vi "updateValues.vi"(8 "error in (no error)":errorcluster, 11 "Rf_Ramp_Action in":refnum<class "Rf_Ramp_Action.lvclass">) -> (0 "error out":errorcluster, 3 "Rf_Ramp_Action out":refnum<class "Rf_Ramp_Action.lvclass">)   [LabVIEW 2011, in "Views.lvlib" / "ScriptEditor.lvlib" / "Rf_Ramp_Action.lvclass"]
uses:
  Rf_Ramp_Action.lvclass
  Tools/Scripting/ScriptingEvent/ScriptEvents/RfRamp/RfRamp.lvclass
  Rf_Ramp_Action.lvclass/Rf_Ramp_Action.ctl
  Tools/Scripting/ScriptingEvent/ScriptEvent.lvclass
  Tools/Scripting/ScriptingEvent/ScriptEvents/Rf Event/rf.lvclass
  ActionPanel.lvclass
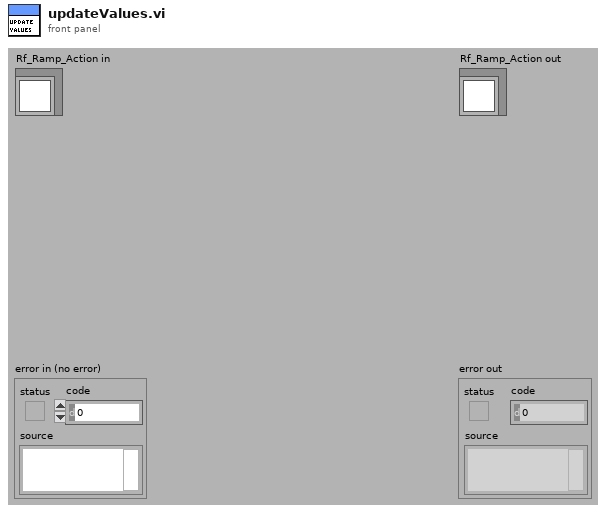
[diagram p1: front panel]
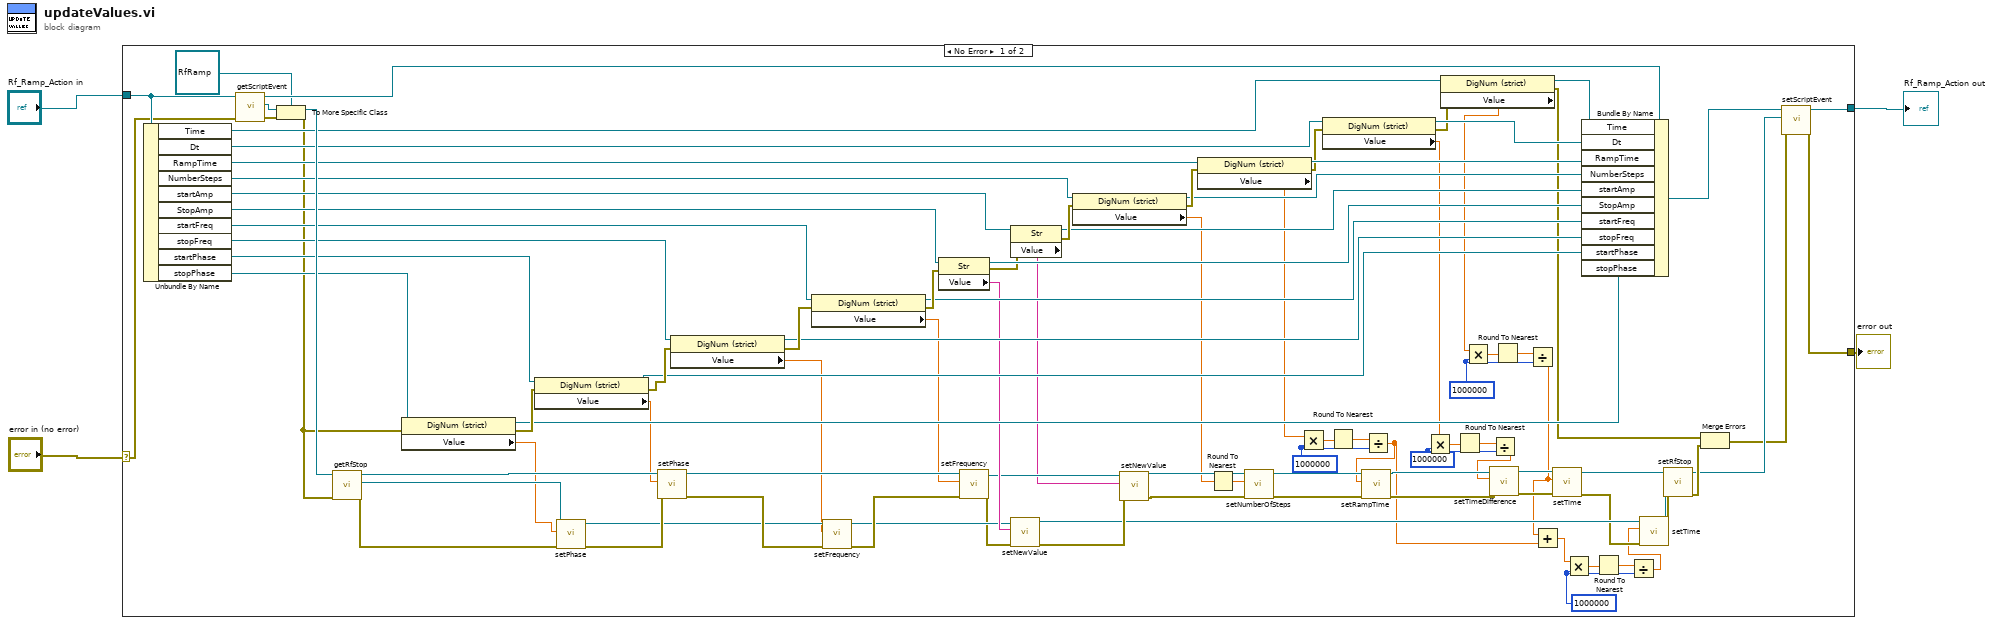
[diagram p0: block diagram]
diagram:
  n1 = case shown="No Error" "error in (no error)" {
    selector: "error in (no error)" -> [w100 w103]
    tunnel: [w27 w103] -> w3
    tunnel: [w29 w102] -> w1
    tunnel: "Rf_Ramp_Action in" -> [w101 w102]
    frame No Error {
      w7 = 1000000
      w12 = 1000000
      w17 = 1000000
      w22 = 1000000
      n2 = Unbundle By Name(w101) -> ("Time"=w67:refnum<vi>, "Dt"=w70:refnum<vi>, "RampTime"=w72:refnum<vi>, "NumberSteps"=w73:refnum<vi>, "startAmp"=w75:refnum<vi>, "StopAmp"=w78:refnum<vi>, "startFreq"=w79:refnum<vi>, "stopFreq"=w80:refnum<vi>, "startPhase"=w81:refnum<vi>, "stopPhase"=w82:refnum<vi>)
      n3 = call "getScriptEvent.vi"("error in (no error)"=w100, "ActionPanel.lvclass in"=w101) -> ("error out"=w84:errorcluster, "ScriptEvent.lvclass"=w86:refnum<class "ScriptEvent.lvclass">, "ActionPanel.lvclass out"=w87:refnum<class "Rf_Ramp_Action.lvclass">)  [unwired: 7 in]
      n4 = To More Specific Class(target class=refnum<class "RfRamp.lvclass"> refnum ("RfRamp out"), reference=w86, error in=w84) -> (specific class reference=w83:refnum<class "RfRamp.lvclass">, error out=w61:errorcluster)
      n5 = call "getRfStop.vi"("error in (no error)"=w61, "RfRamp in"=w83) -> ("error out"=w62:errorcluster, "rfStop"=w66:refnum<class "rf.lvclass">, "RfRamp out"=w65:refnum<class "RfRamp.lvclass">)  [unwired: 7 in]
      n6 = property class="DigNum (strict)"(reference=w82, error in=w61) -> (reference out=w88:refnum<vi>, error out=w89:errorcluster, "Value"=w26:dbl)
      n7 = property class="DigNum (strict)"(reference=w81, error in=w89) -> (reference out=w90:refnum<vi>, error out=w99:errorcluster, "Value"=w64:dbl)
      n8 = call "setPhase.vi"("error in (no error)"=w62, "phase"=w26, "rf in"=w66) -> ("error out"=w63:errorcluster, "rf out"=w57:refnum<class "rf.lvclass">)  [unwired: 7 in]
      n9 = call "setPhase.vi"("error in (no error)"=w63, "phase"=w64, "rf in"=w65) -> ("error out"=w58:errorcluster, "rf out"=w60:refnum<class "RfRamp.lvclass">)  [unwired: 7 in]
      n10 = property class="DigNum (strict)"(reference=w80, error in=w99) -> (reference out=w91:refnum<vi>, error out=w98:errorcluster, "Value"=w56:dbl)
      n11 = property class="DigNum (strict)"(reference=w79, error in=w98) -> (reference out=w92:refnum<vi>, error out=w97:errorcluster, "Value"=w55:dbl)
      n12 = call "setFrequency.vi"("error in (no error)"=w58, "frequency"=w56, "rf in"=w57) -> ("error out"=w59:errorcluster, "rf out"=w53:refnum<class "rf.lvclass">)  [unwired: 7 in]
      n13 = property class="Str"(reference=w78, error in=w97) -> (reference out=w93:refnum<vi>, error out=w76:errorcluster, "Value"=w54:string)
      n14 = call "setFrequency.vi"("error in (no error)"=w59, "frequency"=w55, "rf in"=w60) -> ("error out"=w52:errorcluster, "rf out"=w51:refnum<class "RfRamp.lvclass">)  [unwired: 7 in]
      n15 = property class="Str"(reference=w75, error in=w76) -> (reference out=w74:refnum<vi>, error out=w77:errorcluster, "Value"=w49:string)
      n16 = call "setNewValue.vi"("error in (no error)"=w52, "newValue"=w54, "ScriptEvent.lvclass in"=w53) -> ("error out"=w50:errorcluster, "ScriptEvent.lvclass out"=w39:refnum<class "rf.lvclass">)  [unwired: 7 in]
      n17 = property class="DigNum (strict)"(reference=w73, error in=w77) -> (reference out=w94:refnum<vi>, error out=w96:errorcluster, "Value"=w47:dbl)
      n18 = call "setNewValue.vi"("error in (no error)"=w50, "newValue"=w49, "ScriptEvent.lvclass in"=w51) -> ("error out"=w46:errorcluster, "ScriptEvent.lvclass out"=w48:refnum<class "RfRamp.lvclass">)  [unwired: 7 in]
      n19 = property class="DigNum (strict)"(reference=w72, error in=w96) -> (reference out=w95:refnum<vi>, error out=w71:errorcluster, "Value"=w21:dbl)
      n20 = Round To Nearest(number=w47) -> (nearest integer value=w25:dbl)
      n21 = call "setNumberOfSteps.vi"("error in (no error)"=w46, "NumberOfSteps"=w25, "RfRamp in"=w48) -> ("error out"=w44:errorcluster, "RfRamp out"=w45:refnum<class "RfRamp.lvclass">)  [unwired: 7 in]
      n22 = Multiply(x=w21, y=w22) -> (x*y=w24:dbl)
      n23 = property class="DigNum (strict)"(reference=w70, error in=w71) -> (reference out=w69:refnum<vi>, error out=w43:errorcluster, "Value"=w16:dbl)
      n24 = Round To Nearest(number=w24) -> (nearest integer value=w23:dbl)
      n25 = Divide(x=w23, y=w22) -> (x/y=w20:dbl)
      n26 = call "setRampTime.vi"("error in (no error)"=w44, "rampTime"=w20, "RfRamp in"=w45) -> ("error out"=w36:errorcluster, "RfRamp out"=w37:refnum<class "RfRamp.lvclass">)  [unwired: 7 in]
      n27 = Multiply(x=w16, y=w17) -> (x*y=w19:dbl)
      n28 = property class="DigNum (strict)"(reference=w67, error in=w43) -> (reference out=w68:refnum<vi>, error out=w40:errorcluster, "Value"=w11:dbl)
      n29 = Round To Nearest(number=w19) -> (nearest integer value=w18:dbl)
      n30 = Multiply(x=w11, y=w12) -> (x*y=w14:dbl)
      n31 = Divide(x=w18, y=w17) -> (x/y=w15:dbl)
      n32 = call "setTimeDifference.vi"("error in (no error)"=w36, "time difference"=w15, "ScriptEvent.lvclass in"=w37) -> ("error out"=w41:errorcluster, "ScriptEvent.lvclass out"=w42:refnum<class "RfRamp.lvclass">)  [unwired: 7 in]
      n33 = Round To Nearest(number=w14) -> (nearest integer value=w13:dbl)
      n34 = Divide(x=w13, y=w12) -> (x/y=w10:dbl)
      n35 = Add(x=w10, y=w20) -> (x+y=w6:dbl)
      n36 = call "setTime.vi"("error in (no error)"=w41, "time"=w10, "ScriptEvent.lvclass in"=w42) -> ("error out"=w38:errorcluster, "ScriptEvent.lvclass out"=w35:refnum<class "RfRamp.lvclass">)  [unwired: 7 in]
      n37 = Multiply(x=w6, y=w7) -> (x*y=w9:dbl)
      n38 = Bundle By Name(cluster=w87, "Time"=w68, "Dt"=w69, "RampTime"=w95, "NumberSteps"=w94, "startAmp"=w74, "StopAmp"=w93, "startFreq"=w92, "stopFreq"=w91, "startPhase"=w90, "stopPhase"=w88) -> (w31:refnum<class "Rf_Ramp_Action.lvclass">)
      n39 = Round To Nearest(number=w9) -> (nearest integer value=w8:dbl)
      n40 = Divide(x=w8, y=w7) -> (x/y=w5:dbl)
      n41 = call "setTime.vi"("error in (no error)"=w38, "time"=w5, "ScriptEvent.lvclass in"=w39) -> ("error out"=w33:errorcluster, "ScriptEvent.lvclass out"=w34:refnum<class "rf.lvclass">)  [unwired: 7 in]
      n42 = call "setRfStop.vi"("error in (no error)"=w33, "rfStop"=w34, "RfRamp in"=w35) -> ("error out"=w32:errorcluster, "RfRamp out"=w30:refnum<class "RfRamp.lvclass">)  [unwired: 7 in]
      n43 = Merge Errors(w40, w32) -> (w28:errorcluster)
      n44 = call "setScriptEvent.vi"("error in (no error)"=w28, "ScriptEvent.lvclass"=w30, "ActionPanel.lvclass in"=w31) -> ("error out"=w27:errorcluster, "ActionPanel.lvclass out"=w29:refnum<class "Rf_Ramp_Action.lvclass">)  [unwired: 7 in]
    }
    frame Error {
    }
  }
  "error out" <- w3
  "Rf_Ramp_Action out" <- w1
